vi "impressum.vi"() -> ()   [LabVIEW 2019]
panel:
  out "String":string
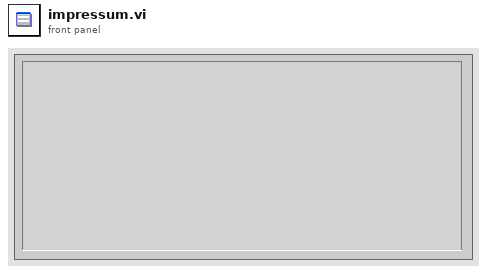
[diagram p1: front panel]
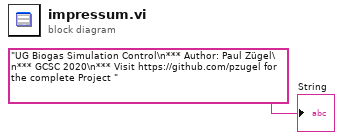
[diagram p0: block diagram]
diagram:
  "String" <- "UG Biogas Simulation Control\n*** Author: Paul Zügel\n*** GCSC 2020\n*** Visit https://github.com/pzugel for the complete Project " ("String")
